vi "PH_IEEE1394Camera.panel.vi"(0 "object ref":refnum<vi>, 5 "error in (no error)":errorcluster) -> (19 "error out":errorcluster)   [LabVIEW 2014, in "PH_IEEE1394Camera.lvlib"]
doc: "This VI is the GUI to control a IEEE1394 Cam.\n\nLicense Agreement for this software:\n\nCopyright (C)\nGesellschaft für Schwerionenforschung, GSI\nPlanckstr. 1\n64291 Darmstadt\nGermany\n\nContact: D.Beck@gsi.de \n\nThis program is free software; you can redistribute it and/or modify it under the terms of the GNU General Public License as published by the Free Software Foundation; either version 2 of the license, or (at your option) any later version.\n\nThis program is distributed in the hope that it will be useful, but WITHOUT ANYW ARRANTY; without even the implied warranty of MERCHANTABILITY or FITNESS FOR A PARTICULAR PURPOSE. See the GNU General License for more details (http://www.gnu.org).\n\nGesellschaft für Schwerionenforschung, GSI\nPlanckstr. 1, 64291 Darmstadt, Germany\nFor all questions and ideas contact: M.Richter@gsi.de, H.Brand@gsi.de or D.Beck@gsi.de.\nLast update: 18-DEC-2002"
uses:
  PH_IEEE1394Camera.lvlib
  PH_Basics/PH_StatusHandler/PH_StatusHandler.GUI element.ctl
  PH_IEEE1394Camera.Cam Attribute.ctl
  <vilib>/vision/driver/IMAQdx.llb/IMAQdx Attribute Type.ctl
  PH_IEEE1394Camera.Cam Details.ctl
  PH_Basics/PH_Cam_BaseClass/PH_Cam_BaseClass.GUI Refs.ctl
  CS_Core/CSObj/CSObj.lvlib
  CS_Core/CSSystem/CSSystemLib/CSSystemLib.lvlib
  PH_Basics/PH_Common/PH_Common.lvlib
  PH_Basics/PH_Cam_BaseClass/PH_Cam_BaseClass.lvlib
  PH_Basics/PH_Class/PH_Class.lvlib
  <vilib>/vision/driver/NI_Vision_Acquisition_Software.lvlib
  PH_Basics/PH_StatusHandler/PH_StatusHandler.lvlib
panel:
  out "PSDB Status":u32(colorbox)=6618880 caption="PSDB"
  out "Status":T1 caption="Camera"
  in  "Tab Control":T2(tab)
  in  "Bit Depth/\nPixel Format":u32(ring) items=["No Info"]
  in  "Start Cam":bool
  in  "Video Mode":u32(ring) items=["Test"]
  in  "Get Histogram":bool
  in  "Logarithmic":bool
  out "Histogram":u32[](graph)
  in  "Gain":dbl
  in  "Brightness":dbl
  in  "Shutter":dbl caption="ms"
  in  "Trigger Timeout":u32=1000 caption="ms"
  in  "Trigger Mode":u32(ring) items=["No Info"]
  in  "Trigger Polarity":u32(ring) items=["No Info"]
  in  "Save Image":bool
  in  "Show Image":bool
  in  "Palette":i32(ring) items=["Grey", "Binary", "Gradient", "Rainbow", "Temperature", "HMH"]
  in  "Scale Factor":i32=50 caption="%" min=30 max=500
  in  "Center of Gravity":bool
  in  "Subtract Background":bool
  in  "Center Cross":bool
  in  "Set ROI to Maximum":bool
  in  "Right":u32
  in  "Left":u32
  in  "Top":u32
  in  "Bottom":u32
  out "Camera Details":T3
  in  "Cam List":u32(ring)
  out "Cam Error":errorcluster
  out "Frames per second":dbl(knob) scale=0.0..30.0 scale format="%.1f"
  in  "Get Frame Rate":bool
  out "Supported Video Modes":T4(array[cluster])
  out "Current Cam Attributes":T5[](array[typedef])
  in  "Boolean Value":bool caption="Value"
  in  "Numeric Value":dbl caption="Value"
  in  "String Value":string caption="Value"
  in  "Attribute to set":u32(ring) caption="Attribute"
  in  "Set Cam Attribute":bool caption="Set"
  in  "Delete":bool
  in  "Exit":bool
  # "PCS"
  # "3.40"
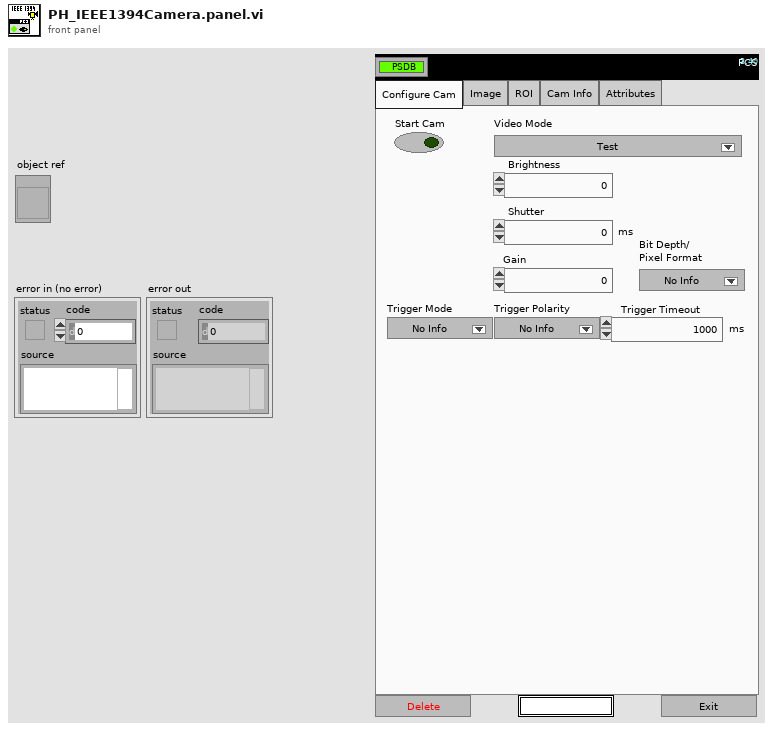
[diagram p1: front panel]
types:
  T1 = typedef "PH_StatusHandler.lvlib/PH_StatusHandler.GUI element.ctl" = u16
  T2 = enum32{"Configure Cam", "Image", "ROI", "Cam Info", "Attributes"}
  T3 = typedef "PH_IEEE1394Camera.lvlib/PH_IEEE1394Camera.Cam Details.ctl" = cluster{"Model":string, "Serial Number":dbl, "Cam name (Machinery)":string, "Bus Type":string}
  T4 = cluster{"Video Mode":u32, "Video Mode Name":string}[]
  T5 = typedef "PH_IEEE1394Camera.lvlib/PH_IEEE1394Camera.Cam Attribute.ctl" = cluster{"Information":cluster{"Type":T6, "Readable":bool, "Writable":bool, "Name":string}, "Num Value":dbl, "String Value":string, "Maximum":dbl, "Minimum":dbl, "Units":string, "Description":string, "EnumStrings[]":string[], "EnumValues[]":u32[], "Boolean Value":bool}
  T6 = typedef "NI_Vision_Acquisition_Software.lvlib/IMAQdx Attribute Type.ctl" = enum32{"U32", "I64", "DBL", "String", "Enum", "Bool", "Command"}
  T7 = typedef "PH_Cam_BaseClass.lvlib/PH_Cam_BaseClass.GUI Refs.ctl" = cluster{"Frame Rate":refnum<vi>, "Get Frame Rate":refnum<vi>, "Show Image":refnum<vi>, "Get Histogram":refnum<vi>, "Mapping":refnum<vi>, "Histogram":refnum<vi>, "Center Cross":refnum<vi>, "Center of Gravity":refnum<vi>, "Scale Factor [%]":refnum<vi>, "Save Image":refnum<vi>, "Palette":refnum<vi>, "Subtract Background":refnum<vi>, "Cam Error":refnum<vi>, "On":refnum<vi>, "Cam List":refnum<vi>}
  T8 = cluster{"Cam Base ClassGui Refs":T7, "PSDB Status":refnum<vi>, "Status":refnum<vi>}
  T9 = typedef "PH_IEEE1394Camera.lvlib/PH_IEEE1394Camera.i attribute.ctl" = cluster{"Gui Refs":cluster{"Brightness":refnum<vi>, "Shutter":refnum<vi>, "Gain":refnum<vi>, "Center of Gravity":refnum<vi>, "Supported Video Modes":refnum<vi>, "Trigger Polarity":refnum<vi>, "Trigger Mode":refnum<vi>, "Trigger Timeout":refnum<vi>, "Bit Depth":refnum<vi>, "Video Mode":refnum<vi>, "Top":refnum<vi>, "Bottom":refnum<vi>, "Left":refnum<vi>, "Right":refnum<vi>, "Set ROI to Maximum":refnum<vi>, "Camera Details":refnum<vi>, "Current Cam Attributes":refnum<vi>, "Attribute to set":refnum<vi>, "Num Value":refnum<vi>, "String Value":refnum<vi>, "Bool Value":refnum<vi>, "Set Cam Attribute":refnum<vi>}, "Cam":cluster{"IMAQ1394 Session":T10, "Camera Details":T3}, "Current Attributes":T5[], "Supported Video Modes ":cluster{"Video Mode":u32, "Video Mode Name":string}[], "Wanted Attributes":cluster{"Name":string, "Num Value":dbl, "String Value":string, "Boolean Value":bool}[], "Cam Attributes":T11}
  T10 = typedef "IMAQdx.ctl" = refnum<k21>
  T11 = typedef "PH_IEEE1394Camera.lvlib/PH_IEEE1394Camera.Relevant Cam Attributes.ctl" = cluster{"Video Mode":cluster{"Name":string, "Index":i32}, "Brightness":cluster{"Name":string, "Index":i32}, "Gain":cluster{"Name":string, "Index":i32}, "Shutter":cluster{"Name":string, "Index":i32}, "Trigger Pol":cluster{"Name":string, "Index":i32}, "Trigger Mode":cluster{"Name":string, "Index":i32}, "Timeout":cluster{"Name":string, "Index":i32}, "Bit Depth":cluster{"Name":string, "Index":i32}, "Pixel Bits":cluster{"Name":string, "Index":i32}, "Pixel Bytes":cluster{"Name":string, "Index":i32}, "Left":cluster{"Name":string, "Index":i32}, "Right":cluster{"Name":string, "Index":i32}, "Top":cluster{"Name":string, "Index":i32}, "Bottom":cluster{"Name":string, "Index":i32}}
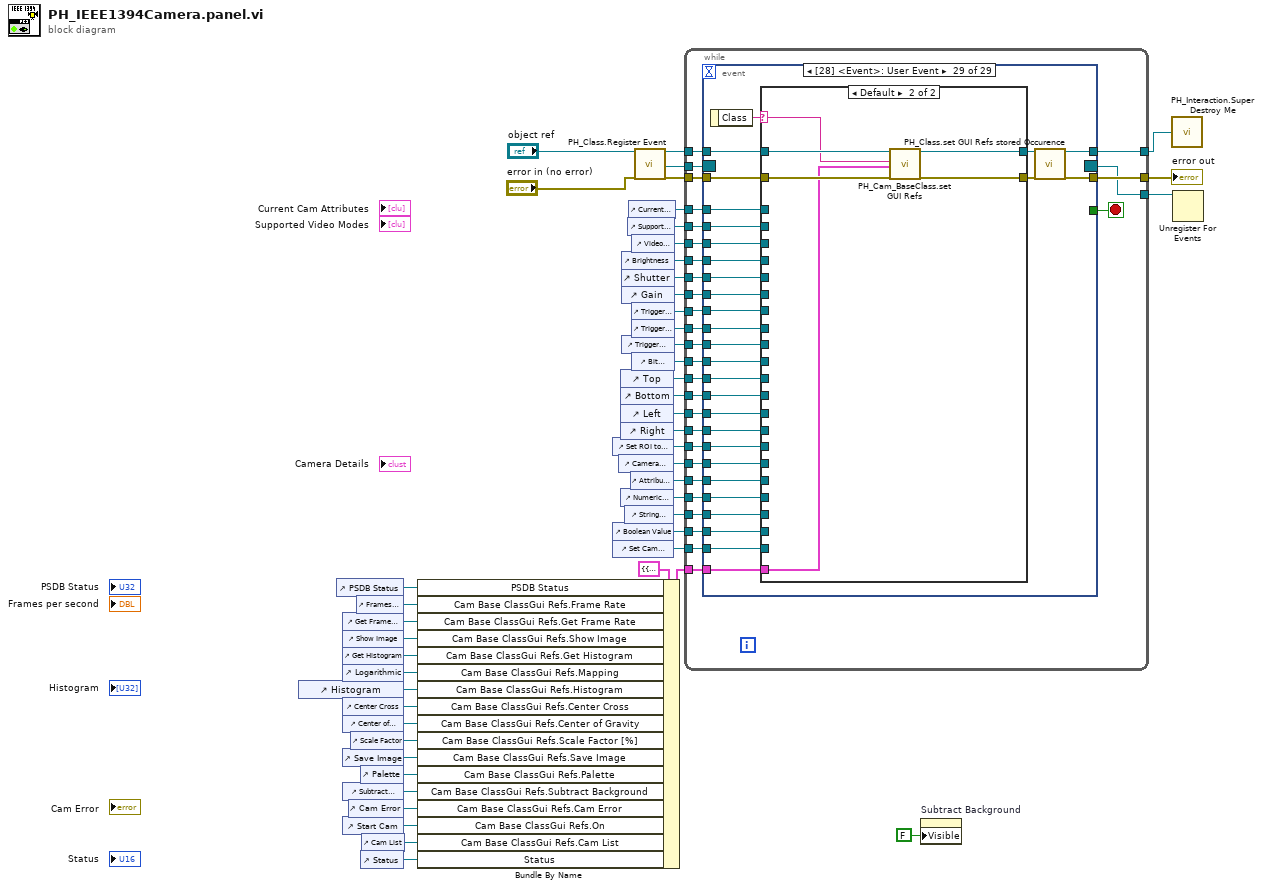
[diagram p0: block diagram]
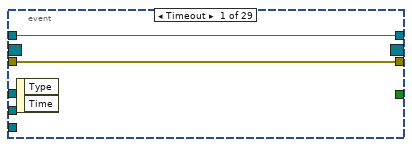
[diagram p2: hidden frame]
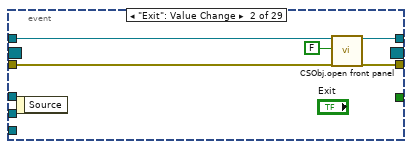
[diagram p3: hidden frame]
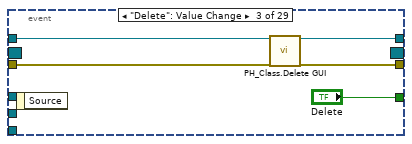
[diagram p4: hidden frame]
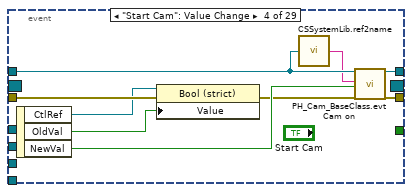
[diagram p5: hidden frame]
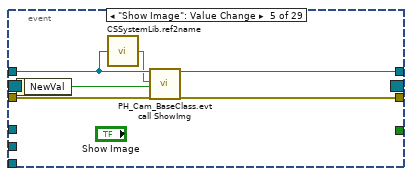
[diagram p6: hidden frame]
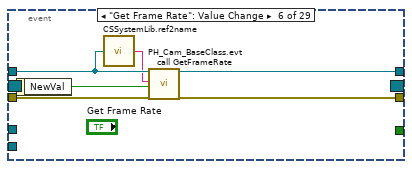
[diagram p7: hidden frame]
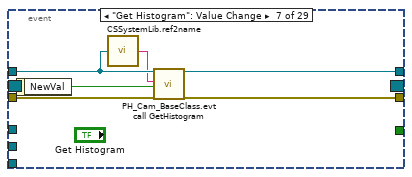
[diagram p8: hidden frame]
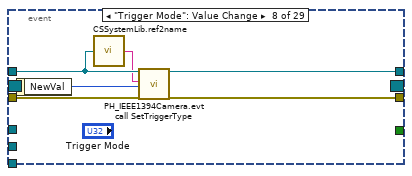
[diagram p9: hidden frame]
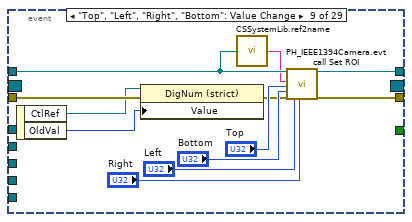
[diagram p10: hidden frame]
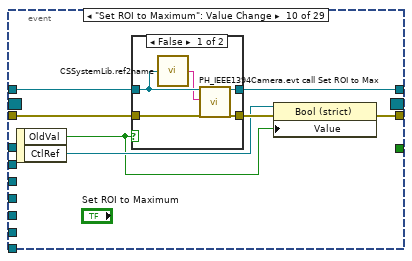
[diagram p11: hidden frame]
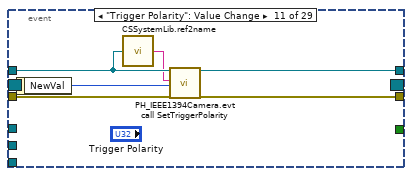
[diagram p13: hidden frame]
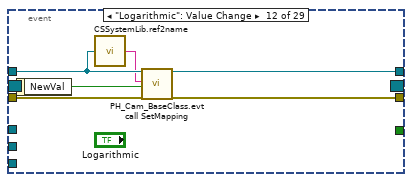
[diagram p14: hidden frame]
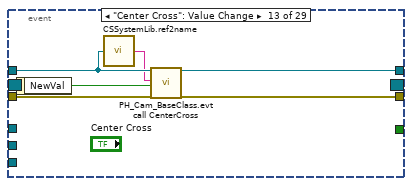
[diagram p15: hidden frame]
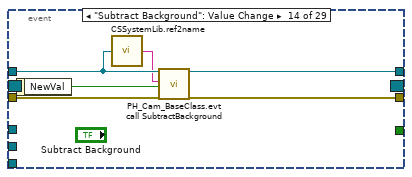
[diagram p16: hidden frame]
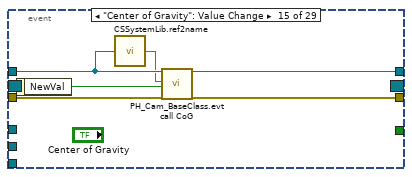
[diagram p17: hidden frame]
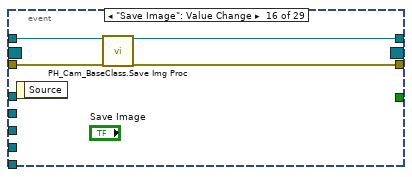
[diagram p18: hidden frame]
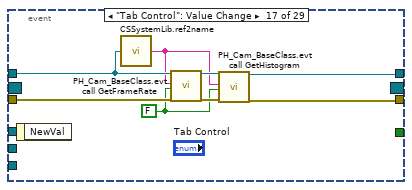
[diagram p19: hidden frame]
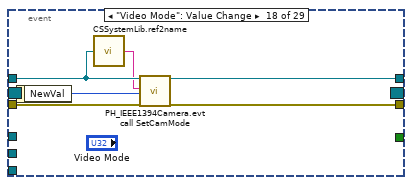
[diagram p20: hidden frame]
diagram:
  n1 = control-ref of="Histogram"() -> (w42:refnum<vi>)
  n2 = control-ref of="PSDB Status"() -> (w3:refnum<vi>)
  n3 = control-ref of="Get Frame Rate"() -> (w46:refnum<vi>)
  n4 = control-ref of="Show Image"() -> (w45:refnum<vi>)
  n5 = control-ref of="Get Histogram"() -> (w44:refnum<vi>)
  n6 = control-ref of="Logarithmic"() -> (w43:refnum<vi>)
  n7 = control-ref of="Center Cross"() -> (w41:refnum<vi>)
  n8 = control-ref of="Center of Gravity"() -> (w39:refnum<vi>)
  n9 = control-ref of="Save Image"() -> (w37:refnum<vi>)
  n10 = control-ref of="Subtract Background"() -> (w40:refnum<vi>)
  n11 = control-ref of="Start Cam"() -> (w33:refnum<vi>)
  n12 = control-ref of="Cam Error"() -> (w34:refnum<vi>)
  n13 = control-ref of="Scale Factor"() -> (w38:refnum<vi>)
  n14 = control-ref of="Frames per second"() -> (w47:refnum<vi>)
  n15 = control-ref of="Palette"() -> (w36:refnum<vi>)
  n16 = control-ref of="Status"() -> (w1:refnum<vi>)
  n17 = control-ref of="Cam List"() -> (w32:refnum<vi>)
  n18 = Bundle By Name(cluster=T8 {"Cam Base ClassGui Refs"={"Frame Rate"=refnum, "Get Frame Rate"=refnum, "Show Image"=refnum, "Get Histogram"=refnum, "Mapping"=refnum, "Histogram"=refnum, "Center Cross"=refnum, "Center of Gravity"=refnum, "Scale Factor [%]"=refnum, "Save Image"=refnum, "Palette"=refnum, "Subtract Background"=refnum, "Cam Error"=refnum, "On"=refnum, "Cam List"=refnum}, "PSDB Status"=refnum, "Status"=refnum} ("GUI Refs to set"), "PSDB Status"=w3, "Cam Base ClassGui Refs.Frame Rate"=w47, "Cam Base ClassGui Refs.Get Frame Rate"=w46, "Cam Base ClassGui Refs.Show Image"=w45, "Cam Base ClassGui Refs.Get Histogram"=w44, "Cam Base ClassGui Refs.Mapping"=w43, "Cam Base ClassGui Refs.Histogram"=w42, "Cam Base ClassGui Refs.Center Cross"=w41, "Cam Base ClassGui Refs.Center of Gravity"=w39, "Cam Base ClassGui Refs.Scale Factor [%]"=w38, "Cam Base ClassGui Refs.Save Image"=w37, "Cam Base ClassGui Refs.Palette"=w36, "Cam Base ClassGui Refs.Subtract Background"=w40, "Cam Base ClassGui Refs.Cam Error"=w34, "Cam Base ClassGui Refs.On"=w33, "Cam Base ClassGui Refs.Cam List"=w32, "Status"=w1) -> (w4:T8)
  n19 = control-ref of="Set ROI to Maximum"() -> (w11:refnum<vi>)
  n20 = control-ref of="Boolean Value"() -> (w6:refnum<vi>)
  n21 = control-ref of="Set Cam Attribute"() -> (w5:refnum<vi>)
  n22 = control-ref of="Camera Details"() -> (w10:refnum<vi>)
  n23 = control-ref of="Top"() -> (w15:refnum<vi>)
  n24 = control-ref of="Bottom"() -> (w14:refnum<vi>)
  n25 = control-ref of="Left"() -> (w13:refnum<vi>)
  n26 = control-ref of="Right"() -> (w12:refnum<vi>)
  n27 = control-ref of="Numeric Value"() -> (w8:refnum<vi>)
  n28 = control-ref of="Brightness"() -> (w22:refnum<vi>)
  n29 = control-ref of="Shutter"() -> (w21:refnum<vi>)
  n30 = control-ref of="Gain"() -> (w20:refnum<vi>)
  n31 = control-ref of="Trigger Timeout"() -> (w17:refnum<vi>)
  n32 = control-ref of="String Value"() -> (w7:refnum<vi>)
  n33 = control-ref of="Supported Video Modes"() -> (w24:refnum<vi>)
  n34 = control-ref of="Current Cam Attributes"() -> (w25:refnum<vi>)
  n35 = control-ref of="Attribute to set"() -> (w9:refnum<vi>)
  n36 = control-ref of="Video Mode"() -> (w23:refnum<vi>)
  n37 = control-ref of="Trigger Mode"() -> (w19:refnum<vi>)
  n38 = control-ref of="Trigger Polarity"() -> (w18:refnum<vi>)
  n39 = control-ref of="Bit Depth/\nPixel Format"() -> (w16:refnum<vi>)
  n40 = call "PH_Class.Register Event.vi"("i ref in"="object ref", "error in (no error)"="error in (no error)") -> ("i ref out"=w31:refnum<vi>, "Event Registration Refnum"=w29:refnum<event-registration>, "error out"=w30:errorcluster)  [unwired: 15 in]
  n41 = while {
    tunnel: w31 -> [w75]
    tunnel: [w74] -> w48
    tunnel: w30 -> [w77]
    tunnel: [w76] -> w49
    tunnel: w29 -> [w73]
    tunnel: [w72] -> w28
    tunnel: w25 -> [w71]
    tunnel: w24 -> [w70]
    tunnel: w23 -> [w69]
    tunnel: w22 -> [w68]
    tunnel: w21 -> [w67]
    tunnel: w20 -> [w66]
    tunnel: w19 -> [w65]
    tunnel: w18 -> [w64]
    tunnel: w17 -> [w63]
    tunnel: w16 -> [w62]
    tunnel: w15 -> [w61]
    tunnel: w14 -> [w60]
    tunnel: w13 -> [w59]
    tunnel: w12 -> [w58]
    tunnel: w11 -> [w57]
    tunnel: w10 -> [w56]
    tunnel: w9 -> [w55]
    tunnel: w8 -> [w54]
    tunnel: w7 -> [w53]
    tunnel: w6 -> [w52]
    tunnel: w5 -> [w51]
    tunnel: w4 -> [w50]
    stop <- w78 stop-if-true
    n42 = event shown="[28] <Event>: User Event" {
      selector: w73 -> [_ _ _ _ _ _ _ _ _ _ _ _ _ _ _ _ _ _ _ _ _ _ _ _ _ _ _ _ _]
      dyn-events: [_ _ _ _ _ _ _ _ _ _ _ _ _ _ _ _ _ _ _ _ _ _ _ _ _ _ _ _ _] -> w72
      timeout: _ -> [_ _ _ _ _ _ _ _ _ _ _ _ _ _ _ _ _ _ _ _ _ _ _ _ _ _ _ _ _]
      tunnel: [_ _ "Delete" _ _ _ _ _ _ _ _ _ _ _ _ _ _ _ _ _ _ _ _ _ _ _ _ _ _] -> w78
      tunnel: w75 -> [w79 w85 w88 w96 w102 w108 w114 w120 w133 w139 w152 w158 w164 w170 w176 w180 w186 w193 w199 w206 w212 w218 w224 w230 w238 w249 w261 w268 w297]
      tunnel: w77 -> [w80 w83 w89 w99 w105 w111 w117 w123 w125 w142 w155 w161 w167 w173 w179 w183 w189 w197 w203 w209 w215 w221 w227 w233 w241 w246 w256 w267 w296]
      tunnel: [w80 w82 w86 w98 w104 w110 w116 w122 w135 w138 w154 w160 w166 w172 w178 w182 w187 w195 w201 w207 w213 w219 w225 w231 w239 w250 w262 w264 w292] -> w76
      tunnel: [w79 w81 w87 w97 w103 w109 w115 w121 w134 w140 w153 w159 w165 w171 w177 w181 w190 w196 w202 w208 w214 w220 w226 w232 w240 w251 w263 w266 w294] -> w74
      tunnel: w71 -> [_ _ _ _ _ _ _ _ _ _ _ _ _ _ _ _ _ _ _ _ _ _ _ _ _ _ _ _ w290]
      tunnel: w70 -> [_ _ _ _ _ _ _ _ _ _ _ _ _ _ _ _ _ _ _ _ _ _ _ _ _ _ _ _ w289]
      tunnel: w69 -> [_ _ _ _ _ _ _ _ _ _ _ _ _ _ _ _ _ _ _ _ _ _ _ _ _ _ _ _ w288]
      tunnel: w68 -> [_ _ _ _ _ _ _ _ _ _ _ _ _ _ _ _ _ _ _ _ _ _ _ _ _ _ _ _ w287]
      tunnel: w67 -> [_ _ _ _ _ _ _ _ _ _ _ _ _ _ _ _ _ _ _ _ _ _ _ _ _ _ _ _ w286]
      tunnel: w66 -> [_ _ _ _ _ _ _ _ _ _ _ _ _ _ _ _ _ _ _ _ _ _ _ _ _ _ _ _ w285]
      tunnel: w65 -> [_ _ _ _ _ _ _ _ _ _ _ _ _ _ _ _ _ _ _ _ _ _ _ _ _ _ _ _ w284]
      tunnel: w64 -> [_ _ _ _ _ _ _ _ _ _ _ _ _ _ _ _ _ _ _ _ _ _ _ _ _ _ _ _ w283]
      tunnel: w63 -> [_ _ _ _ _ _ _ _ _ _ _ _ _ _ _ _ _ _ _ _ _ _ _ _ _ _ _ _ w282]
      tunnel: w62 -> [_ _ _ _ _ _ _ _ _ _ _ _ _ _ _ _ _ _ _ _ _ _ _ _ _ _ _ _ w281]
      tunnel: w61 -> [_ _ _ _ _ _ _ _ _ _ _ _ _ _ _ _ _ _ _ _ _ _ _ _ _ _ _ _ w280]
      tunnel: w60 -> [_ _ _ _ _ _ _ _ _ _ _ _ _ _ _ _ _ _ _ _ _ _ _ _ _ _ _ _ w279]
      tunnel: w59 -> [_ _ _ _ _ _ _ _ _ _ _ _ _ _ _ _ _ _ _ _ _ _ _ _ _ _ _ _ w278]
      tunnel: w58 -> [_ _ _ _ _ _ _ _ _ _ _ _ _ _ _ _ _ _ _ _ _ _ _ _ _ _ _ _ w277]
      tunnel: w57 -> [_ _ _ _ _ _ _ _ _ _ _ _ _ _ _ _ _ _ _ _ _ _ _ _ _ _ _ _ w276]
      tunnel: w56 -> [_ _ _ _ _ _ _ _ _ _ _ _ _ _ _ _ _ _ _ _ _ _ _ _ _ _ _ _ w275]
      tunnel: w55 -> [_ _ _ _ _ _ _ _ _ _ _ _ _ _ _ _ _ _ _ _ _ _ _ _ _ _ _ _ w274]
      tunnel: w54 -> [_ _ _ _ _ _ _ _ _ _ _ _ _ _ _ _ _ _ _ _ _ _ _ _ _ _ _ _ w273]
      tunnel: w53 -> [_ _ _ _ _ _ _ _ _ _ _ _ _ _ _ _ _ _ _ _ _ _ _ _ _ _ _ _ w272]
      tunnel: w52 -> [_ _ _ _ _ _ _ _ _ _ _ _ _ _ _ _ _ _ _ _ _ _ _ _ _ _ _ _ w271]
      tunnel: w51 -> [_ _ _ _ _ _ _ _ _ _ _ _ _ _ _ _ _ _ _ _ _ _ _ _ _ _ _ _ w270]
      tunnel: w50 -> [_ _ _ _ _ _ _ _ _ _ _ _ _ _ _ _ _ _ _ _ _ _ _ _ _ _ _ _ w269]
      event Timeout {
        n43 = event-data() -> ()  [unwired: 1 in, 2 out]
      }
      event "Exit": Value Change {
        n44 = event-data() -> ()  [unwired: 1 in, 1 out]
        n45 = call "CSObj.open front panel.vi"("i ref in"=w85, "frontPanelOpen"=FALSE ("front panel open"), "error in (no error)"=w83) -> ("i ref out"=w81:refnum<vi>, "error out"=w82:errorcluster)  [unwired: 15 in]
      }
      event "Delete": Value Change {
        n46 = event-data() -> ()  [unwired: 1 in, 1 out]
        n47 = call "PH_Class.Delete GUI.vi"("VI in"=w88, "error in (no error)"=w89) -> ("VI out"=w87:refnum<vi>, "error out"=w86:errorcluster)  [unwired: 16 in]
      }
      event "Start Cam": Value Change {
        n48 = event-data() -> ("CtlRef"=w92:refnum<vi>, "OldVal"=w91:bool, "NewVal"=w94:bool)  [unwired: 1 in]
        n49 = property class="Bool (strict)"(reference=w92, error in=w99, "Value"=w91) -> (error out=w93:errorcluster)  [unwired: 1 out]
        n50 = call "CSSystemLib.ref2name.vi"("obj refnum"=w96) -> ("name"=w95:string)
        n51 = call "PH_Cam_BaseClass.evt Cam on.vi"("i ref in"=w96, "Instance"=w95, "Cam on"=w94, "error in (no error)"=w93) -> ("i ref out"=w97:refnum<vi>, "error out"=w98:errorcluster)  [unwired: 14 in]
      }
      event "Show Image": Value Change {
        n52 = event-data() -> ("NewVal"=w100:bool)  [unwired: 1 in]
        n53 = call "CSSystemLib.ref2name.vi"("obj refnum"=w102) -> ("name"=w101:string)
        n54 = call "PH_Cam_BaseClass.evt call ShowImg.vi"("i ref in"=w102, "Instance"=w101, "Start Cam"=w100, "error in (no error)"=w105) -> ("i ref out"=w103:refnum<vi>, "error out"=w104:errorcluster)  [unwired: 14 in]
      }
      event "Get Frame Rate": Value Change {
        n55 = event-data() -> ("NewVal"=w106:bool)  [unwired: 1 in]
        n56 = call "CSSystemLib.ref2name.vi"("obj refnum"=w108) -> ("name"=w107:string)
        n57 = call "PH_Cam_BaseClass.evt call GetFrameRate.vi"("i ref in"=w108, "Instance"=w107, "Get Frame Rate"=w106, "error in (no error)"=w111) -> ("i ref out"=w109:refnum<vi>, "error out"=w110:errorcluster)  [unwired: 14 in]
      }
      event "Get Histogram": Value Change {
        n58 = event-data() -> ("NewVal"=w112:bool)  [unwired: 1 in]
        n59 = call "CSSystemLib.ref2name.vi"("obj refnum"=w114) -> ("name"=w113:string)
        n60 = call "PH_Cam_BaseClass.evt call GetHistogram.vi"("i ref in"=w114, "Instance"=w113, "Get Histogram"=w112, "error in (no error)"=w117) -> ("i ref out"=w115:refnum<vi>, "error out"=w116:errorcluster)  [unwired: 14 in]
      }
      event "Trigger Mode": Value Change {
        n61 = event-data() -> ("NewVal"=w118:u32)  [unwired: 1 in]
        n62 = call "CSSystemLib.ref2name.vi"("obj refnum"=w120) -> ("name"=w119:string)
        n63 = call "PH_IEEE1394Camera.evt call SetTriggerType.vi"("i ref in"=w120, "Instance"=w119, "Trigger Mode"=w118, "error in (no error)"=w123) -> ("i ref out"=w121:refnum<vi>, "error out"=w122:errorcluster)  [unwired: 14 in]
      }
      event "Top", "Left", "Right", "Bottom": Value Change {
        n64 = event-data() -> ("CtlRef"=w124:refnum<vi>, "OldVal"=w126:u32)  [unwired: 1 in]
        n65 = property class="DigNum (strict)"(reference=w124, error in=w125, "Value"=w126) -> (error out=w127:errorcluster)  [unwired: 1 out]
        n66 = call "CSSystemLib.ref2name.vi"("obj refnum"=w133) -> ("name"=w132:string)
        n67 = call "PH_IEEE1394Camera.evt call Set ROI.vi"("i ref in"=w133, "Instance"=w132, "Top"="Top", "Bottom"="Bottom", "error in (no error)"=w127, "Left"="Left", "Right"="Right") -> ("i ref out"=w134:refnum<vi>, "error out"=w135:errorcluster)  [unwired: 11 in]
      }
      event "Set ROI to Maximum": Value Change {
        n68 = event-data() -> ("OldVal"=w136:bool, "CtlRef"=w137:refnum<vi>)  [unwired: 1 in]
        n69 = case shown="False" w136 {
          tunnel: w142 -> [w147 w148]
          tunnel: [w146 w148] -> w141
          tunnel: [w145 w149] -> w140
          tunnel: w139 -> [w144 w149]
          frame False {
            n70 = call "CSSystemLib.ref2name.vi"("obj refnum"=w144) -> ("name"=w143:string)
            n71 = call "PH_IEEE1394Camera.evt call Set ROI to Max.vi"("i ref in"=w144, "Instance"=w143, "error in (no error)"=w147) -> ("i ref out"=w145:refnum<vi>, "error out"=w146:errorcluster)  [unwired: 15 in]
          }
          frame True {
          }
        }
        n72 = property class="Bool (strict)"(reference=w137, error in=w141, "Value"=w136) -> (error out=w138:errorcluster)  [unwired: 1 out]
      }
      event "Trigger Polarity": Value Change {
        n73 = event-data() -> ("NewVal"=w150:u32)  [unwired: 1 in]
        n74 = call "CSSystemLib.ref2name.vi"("obj refnum"=w152) -> ("name"=w151:string)
        n75 = call "PH_IEEE1394Camera.evt call SetTriggerPolarity.vi"("i ref in"=w152, "Instance"=w151, "Trigger Polarity"=w150, "error in (no error)"=w155) -> ("i ref out"=w153:refnum<vi>, "error out"=w154:errorcluster)  [unwired: 14 in]
      }
      event "Logarithmic": Value Change {
        n76 = event-data() -> ("NewVal"=w156:bool)  [unwired: 1 in]
        n77 = call "CSSystemLib.ref2name.vi"("obj refnum"=w158) -> ("name"=w157:string)
        n78 = call "PH_Cam_BaseClass.evt call SetMapping.vi"("i ref in"=w158, "Instance"=w157, "Get Histogram"=w156, "error in (no error)"=w161) -> ("i ref out"=w159:refnum<vi>, "error out"=w160:errorcluster)  [unwired: 14 in]
      }
      event "Center Cross": Value Change {
        n79 = event-data() -> ("NewVal"=w162:bool)  [unwired: 1 in]
        n80 = call "CSSystemLib.ref2name.vi"("obj refnum"=w164) -> ("name"=w163:string)
        n81 = call "PH_Cam_BaseClass.evt call CenterCross.vi"("i ref in"=w164, "Instance"=w163, "Center Cross"=w162, "error in (no error)"=w167) -> ("i ref out"=w165:refnum<vi>, "error out"=w166:errorcluster)  [unwired: 14 in]
      }
      event "Subtract Background": Value Change {
        n82 = event-data() -> ("NewVal"=w168:bool)  [unwired: 1 in]
        n83 = call "CSSystemLib.ref2name.vi"("obj refnum"=w170) -> ("name"=w169:string)
        n84 = call "PH_Cam_BaseClass.evt call SubtractBackground.vi"("i ref in"=w170, "Instance"=w169, "Subtract Background"=w168, "error in (no error)"=w173) -> ("i ref out"=w171:refnum<vi>, "error out"=w172:errorcluster)  [unwired: 14 in]
      }
      event "Center of Gravity": Value Change {
        n85 = event-data() -> ("NewVal"=w174:bool)  [unwired: 1 in]
        n86 = call "CSSystemLib.ref2name.vi"("obj refnum"=w176) -> ("name"=w175:string)
        n87 = call "PH_Cam_BaseClass.evt call CoG.vi"("i ref in"=w176, "Instance"=w175, "Set CoG"=w174, "error in (no error)"=w179) -> ("i ref out"=w177:refnum<vi>, "error out"=w178:errorcluster)  [unwired: 14 in]
      }
      event "Save Image": Value Change {
        n88 = event-data() -> ()  [unwired: 1 in, 1 out]
        n89 = call "PH_Cam_BaseClass.Save Img Proc.vi"("VI in"=w180, "error in (no error)"=w183) -> ("VI out"=w181:refnum<vi>, "error out"=w182:errorcluster)  [unwired: 16 in]
      }
      event "Tab Control": Value Change {
        w184 = FALSE
        n90 = event-data() -> ()  [unwired: 1 in, 1 out]
        n91 = call "CSSystemLib.ref2name.vi"("obj refnum"=w186) -> ("name"=w185:string)
        n92 = call "PH_Cam_BaseClass.evt call GetFrameRate.vi"("i ref in"=w186, "Instance"=w185, "Get Frame Rate"=w184, "error in (no error)"=w189) -> ("i ref out"=w191:refnum<vi>, "error out"=w188:errorcluster)  [unwired: 14 in]
        n93 = call "PH_Cam_BaseClass.evt call GetHistogram.vi"("i ref in"=w191, "Instance"=w185, "Get Histogram"=w184, "error in (no error)"=w188) -> ("i ref out"=w190:refnum<vi>, "error out"=w187:errorcluster)  [unwired: 14 in]
      }
      event "Video Mode": Value Change {
        n94 = event-data() -> ("NewVal"=w194:u32)  [unwired: 1 in]
        n95 = call "CSSystemLib.ref2name.vi"("obj refnum"=w193) -> ("name"=w192:string)
        n96 = call "PH_IEEE1394Camera.evt call SetCamMode.vi"("i ref in"=w193, "Instance"=w192, "Select Video Mode"=w194, "error in (no error)"=w197) -> ("i ref out"=w196:refnum<vi>, "error out"=w195:errorcluster)  [unwired: 14 in]
      }
      event "Bit Depth/\nPixel Format": Value Change {
        n97 = event-data() -> ("NewVal"=w200:u32)  [unwired: 1 in]
        n98 = call "CSSystemLib.ref2name.vi"("obj refnum"=w199) -> ("name"=w198:string)
        n99 = call "PH_IEEE1394Camera.evt call SetBitDepth.vi"("i ref in"=w199, "Instance"=w198, "Bit Depth"=w200, "error in (no error)"=w203) -> ("i ref out"=w202:refnum<vi>, "error out"=w201:errorcluster)  [unwired: 14 in]
      }
      event "Brightness": Value Change {
        n100 = event-data() -> ("NewVal"=w204:dbl)  [unwired: 1 in]
        n101 = call "CSSystemLib.ref2name.vi"("obj refnum"=w206) -> ("name"=w205:string)
        n102 = call "PH_IEEE1394Camera.evt call SetBrightness.vi"("i ref in"=w206, "Instance"=w205, "Brightness"=w204, "error in (no error)"=w209) -> ("i ref out"=w208:refnum<vi>, "error out"=w207:errorcluster)  [unwired: 14 in]
      }
      event "Shutter": Value Change {
        n103 = event-data() -> ("NewVal"=w210:dbl)  [unwired: 1 in]
        n104 = call "CSSystemLib.ref2name.vi"("obj refnum"=w212) -> ("name"=w211:string)
        n105 = call "PH_IEEE1394Camera.evt call SetShutter.vi"("i ref in"=w212, "Instance"=w211, "Shutter"=w210, "error in (no error)"=w215) -> ("i ref out"=w214:refnum<vi>, "error out"=w213:errorcluster)  [unwired: 14 in]
      }
      event "Gain": Value Change {
        n106 = event-data() -> ("NewVal"=w216:dbl)  [unwired: 1 in]
        n107 = call "CSSystemLib.ref2name.vi"("obj refnum"=w218) -> ("name"=w217:string)
        n108 = call "PH_IEEE1394Camera.evt call SetGain.vi"("i ref in"=w218, "Instance"=w217, "Gain"=w216, "error in (no error)"=w221) -> ("i ref out"=w220:refnum<vi>, "error out"=w219:errorcluster)  [unwired: 14 in]
      }
      event "Trigger Timeout": Value Change {
        n109 = event-data() -> ("NewVal"=w222:u32)  [unwired: 1 in]
        n110 = call "CSSystemLib.ref2name.vi"("obj refnum"=w224) -> ("name"=w223:string)
        n111 = call "PH_IEEE1394Camera.evt call SetTimeout.vi"("i ref in"=w224, "Instance"=w223, "TO [ms]"=w222, "error in (no error)"=w227) -> ("i ref out"=w226:refnum<vi>, "error out"=w225:errorcluster)  [unwired: 14 in]
      }
      event "Palette": Value Change {
        n112 = event-data() -> ("NewVal"=w228:i32)  [unwired: 1 in]
        n113 = call "CSSystemLib.ref2name.vi"("obj refnum"=w230) -> ("name"=w229:string)
        n114 = call "PH_Cam_BaseClass.evt call SetPalette.vi"("i ref in"=w230, "Instance"=w229, "Palette"=w228, "error in (no error)"=w233) -> ("i ref out"=w232:refnum<vi>, "error out"=w231:errorcluster)  [unwired: 14 in]
      }
      event "Scale Factor": Value Change {
        n115 = event-data() -> ("NewVal"=w235:i32)  [unwired: 1 in]
        n116 = call "CSSystemLib.ref2name.vi"("obj refnum"=w238) -> ("name"=w237:string)
        n117 = Divide(x=w235, y=100) -> (x/y=w234:dbl)
        n118 = call "PH_Cam_BaseClass.evt call SetScaleFactor.vi"("i ref in"=w238, "Instance"=w237, "Scale Factor [%]"=w234, "error in (no error)"=w241) -> ("i ref out"=w240:refnum<vi>, "error out"=w239:errorcluster)  [unwired: 14 in]
      }
      event "Cam List": Value Change {
        n119 = event-data() -> ("CtlRef"=w247:refnum<vi>)  [unwired: 1 in]
        n120 = property class="Ring (strict)"(reference=w247, error in=w246) -> (error out=w245:errorcluster, "Strings []"=w244:string[], "Value"=w242:u32)  [unwired: 1 out]
        n121 = call "CSSystemLib.ref2name.vi"("obj refnum"=w249) -> ("name"=w248:string)
        n122 = Index Array(array=w244, index=w242) -> (element=w243:string)
        n123 = call "PH_Cam_BaseClass.evt call Connect.vi"("i ref in"=w249, "Instance"=w248, "Cam Name"=w243, "error in (no error)"=w245) -> ("i ref out"=w251:refnum<vi>, "error out"=w250:errorcluster)  [unwired: 14 in]
      }
      event "Set Cam Attribute": Value Change {
        n124 = event-data() -> ()  [unwired: 1 in, 1 out]
        n125 = property on="Attribute to set" class="Ring (strict)"(error in=w256) -> (error out=w255:errorcluster, "Strings []"=w254:string[], "Value"=w253:u32)  [unwired: 1 in, 1 out]
        n126 = call "CSSystemLib.ref2name.vi"("obj refnum"=w261) -> ("name"=w260:string)
        n127 = Index Array(array=w254, index=w253) -> (element=w252:string)
        n128 = call "PH_IEEE1394Camera.evt CamAttr Write.vi"("i ref in"=w261, "Instance"=w260, "Set Num"="Numeric Value", "Set String"="String Value", "Set Bool"="Boolean Value", "error in (no error)"=w255, "Attribute Name"=w252) -> ("i ref out"=w263:refnum<vi>, "error out"=w262:errorcluster)  [unwired: 11 in]
      }
      event "Attribute to set": Value Change {
        n129 = event-data() -> ("NewVal"=w265:u32)  [unwired: 1 in]
        n130 = call "PH_IEEE1394Camera.set Visibility of Cam Attribute Value Set Knobs.vi"("VI in"=w268, "Index of selected Attribute"=w265, "error in (no error)"=w267) -> ("VI out"=w266:refnum<vi>, "error out"=w264:errorcluster)  [unwired: 15 in]
      }
      event User Event {
        n131 = event-data() -> ("Class"=w291:string)  [unwired: 1 in]
        n132 = case shown="Default" w291 {
          selector: w291 -> [_ w329]
          tunnel: w297 -> [w322 w333]
          tunnel: w296 -> [w321 w332]
          tunnel: [w320 w331] -> w295
          tunnel: [w319 w330] -> w293
          tunnel: w290 -> [w318 _]
          tunnel: w289 -> [w317 _]
          tunnel: w288 -> [w316 _]
          tunnel: w287 -> [w300 _]
          tunnel: w286 -> [w299 _]
          tunnel: w285 -> [w298 _]
          tunnel: w284 -> [w315 _]
          tunnel: w283 -> [w314 _]
          tunnel: w282 -> [w313 _]
          tunnel: w281 -> [w312 _]
          tunnel: w280 -> [w311 _]
          tunnel: w279 -> [w310 _]
          tunnel: w278 -> [w309 _]
          tunnel: w277 -> [w308 _]
          tunnel: w276 -> [w307 _]
          tunnel: w275 -> [w306 _]
          tunnel: w274 -> [w305 _]
          tunnel: w273 -> [w304 _]
          tunnel: w272 -> [w303 _]
          tunnel: w271 -> [w302 _]
          tunnel: w270 -> [w301 _]
          tunnel: w269 -> [_ w328]
          frame "PH_IEEE1394Camera" {
            n133 = call "PH_IEEE1394Camera.get data to modify.vi"("i ref in"=w322, "ms timeout (10000)"=-1, "error in (no error)"=w321) -> ("i ref out"=w327:refnum<vi>, "i attribute"=w324:T9, "error out"=w326:errorcluster)  [unwired: 13 in, 1 out]
            n134 = Bundle By Name(cluster=w324, "Gui Refs.Current Cam Attributes"=w318, "Gui Refs.Supported Video Modes"=w317, "Gui Refs.Video Mode"=w316, "Gui Refs.Brightness"=w300, "Gui Refs.Shutter"=w299, "Gui Refs.Gain"=w298, "Gui Refs.Trigger Mode"=w315, "Gui Refs.Trigger Polarity"=w314, "Gui Refs.Trigger Timeout"=w313, "Gui Refs.Bit Depth"=w312, "Gui Refs.Top"=w311, "Gui Refs.Bottom"=w310, "Gui Refs.Left"=w309, "Gui Refs.Right"=w308, "Gui Refs.Set ROI to Maximum"=w307, "Gui Refs.Camera Details"=w306, "Gui Refs.Attribute to set"=w305, "Gui Refs.Num Value"=w304, "Gui Refs.String Value"=w303, "Gui Refs.Bool Value"=w302, "Gui Refs.Set Cam Attribute"=w301) -> (w323:T9)
            n135 = call "PH_IEEE1394Camera.set modified data.vi"("i ref in"=w327, "i attribute"=w323, "error in (no error)"=w326) -> ("i ref out"=w320:refnum<vi>, "error out"=w319:errorcluster)  [unwired: 15 in]
          }
          frame Default {
            n136 = call "PH_Cam_BaseClass.set GUI Refs.vi"("VI in"=w333, "Class"=w329, "GUI Refs to set"=w328, "error in (no error)"=w332) -> ("VI out"=w331:refnum<vi>, "error out"=w330:errorcluster)  [unwired: 14 in]
          }
        }
        n137 = call "PH_Class.set GUI Refs stored Occurence.vi"("i ref in"=w295, "error in (no error)"=w293) -> ("i ref out"=w294:refnum<vi>, "error out"=w292:errorcluster)  [unwired: 16 in]
      }
    }
  }
  "error out" <- w49
  n138 = property on="Subtract Background" class="Bool (strict)"("Visible"=FALSE) -> ()  [unwired: 2 in, 2 out]
  n139 = call "PH_Interaction.Super Destroy Me.vi"("i ref out"=w48) -> ()
  n140 = Unregister For Events(event registration refnum=w28) -> ()  [unwired: 1 in, 1 out]
